vi "Gas_Release_Control.vi"(5 "Extra Commands":string, 6 "Density Ratio":string="Carrier 1 only", 7 "Strength (% by volume)":dbl format="%.3f", 8 "Stack flowrate (l/min)":dbl format="%.2f", 9 "Source Status":T2) -> (0 "error out":errorcluster, 1 "Flowrates (kg/min)":dbl[](array[numeric]) format="%.2f", 2 "Source Est Time (s)":dbl, 3 "Flowrates Achieved?":bool)   [LabVIEW 2012]
uses:
  ADAM Controls/Client_Source_Status.ctl
  ADAM Controls/Client_Source.ctl
  ADAM Controls/Channel_names.ctl
  ADAM Controls/Module_type_ADAM.ctl
  ADAM Controls/Calib_type_ADAM.ctl
  ADAM Controls/Channel_State.ctl
  ADAM Controls/Ch_description_ADAM.ctl
  ADAM Controls/Function_ADAM.ctl
  ADAM Controls/Address.ctl
  ADAM Controls/Update_scan_value.ctl
  Anemometry/Anemometry Sub Vis/Controls/In_Range.ctl
  Anemometry/Anemometry Sub Vis/Globals/Preference_global.vi
  Anemometry/Anemometry Sub Vis/Globals/Extra_Commands_Global.vi
panel:
  out "Error String":string
  out "Currently on":T1=enum."Get Source Clients"
  out "Status of other Clients":string[](array[string])
  out "Source already correct?":bool
  out "No Other Clients are Using Source?":bool
  out "Source Clients":string[](array[string])
  # "-Carrier 1 only\n-Carrier 2 only\n-Enter Ratio"
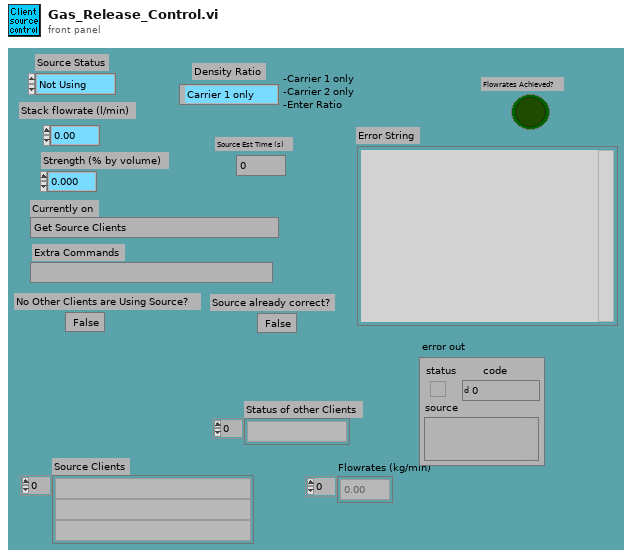
[diagram p1: front panel]
types:
  T1 = typedef "Client_Source.ctl" = enum16{"Start", "Get Source Clients", "Has this client liberty to control the source?", "Declare not using, other client already waiting", "Is the Source already correct?", "Declare waiting, other client is still using", "Control Hi-Tec", "Were the Hi-tecs able to achieve the flowrates?", "Declare source status", "Wait for source to Establish"}
  T2 = typedef "Client_Source_Status.ctl" = enum16{"Not Using", "Using", "Must Have"}
  T3 = typedef "Channel_names.ctl" = enum16{"Active Only", "Active + Off", "All Channels"}
  T4 = typedef "Ch_description_ADAM.ctl" = cluster{"Ch Name":string, "Type":T5, "Function":T6, "Ch State":T7, "Calibration type":T8, "A":dbl, "B":dbl, "C":dbl, "D":dbl, "Comments":string, "Address":T9, "String":string, "Duty":u16}
  T5 = typedef "Module_type_ADAM.ctl" = string
  T6 = typedef "Function_ADAM.ctl" = enum16{"Analogue Input", "Digital Input", "Event counter", "Event rate", "Analogue Output", "Digital Output", "Relay Output"}
  T7 = typedef "Channel_State.ctl" = enum16{"On", "Off", "Always On", "Always Off"}
  T8 = typedef "Calib_type_ADAM.ctl" = enum16{"Raw", "Bx + A", "Cx^2 + Bx + A", "Dx^3 + Cx^2 + Bx + A", "In Band", "Hi-Tec Q", "Hi-Tec M_dot", "Text"}
  T9 = typedef "Address.ctl" = cluster{"Main":i32, "Ch.":i32, "Sub":i32, "Port Name":string}
  T10 = typedef "Update_scan_value.ctl" = cluster{"Channel Name":string, "New Value":dbl}
  T11 = typedef "In_Range.ctl" = enum16{"%", "±", "% & ±"}
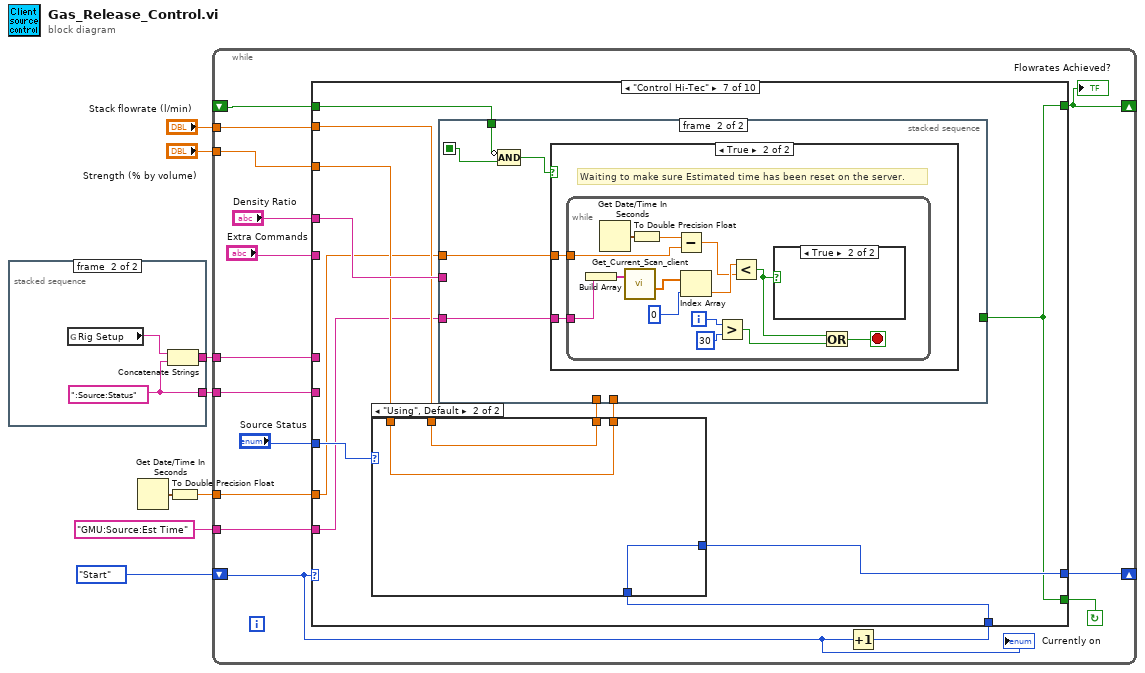
[diagram p0: block diagram]
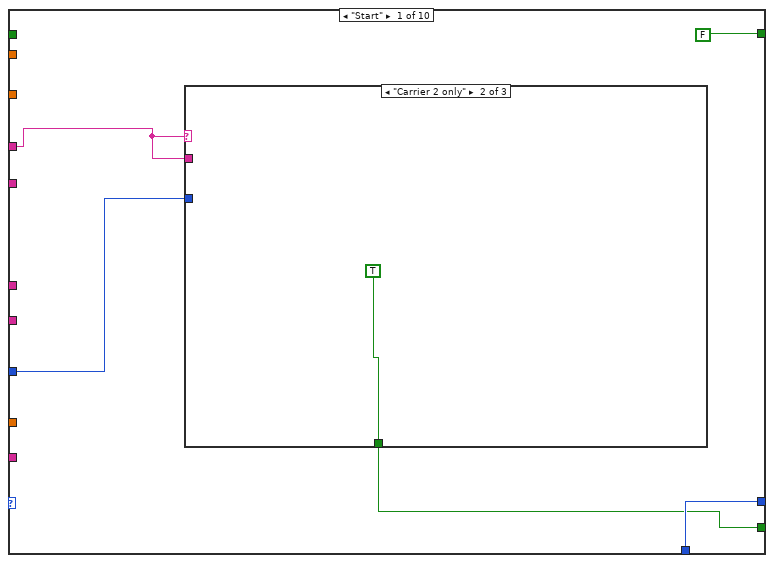
[diagram p2: hidden frame]
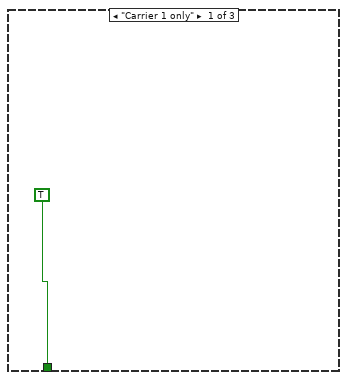
[diagram p3: hidden frame]
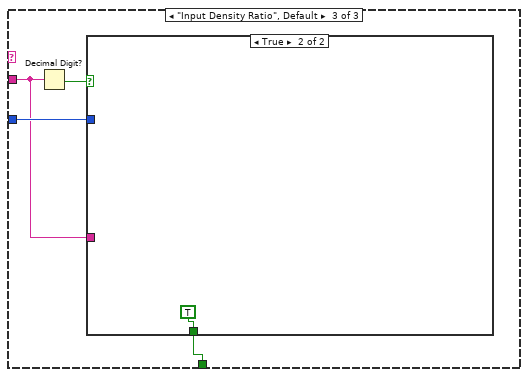
[diagram p4: hidden frame]
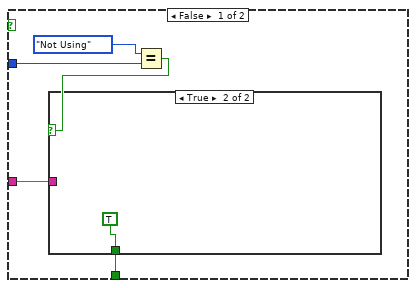
[diagram p5: hidden frame]
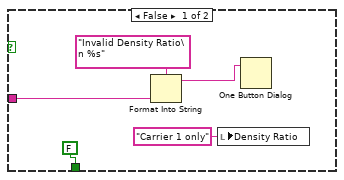
[diagram p6: hidden frame]
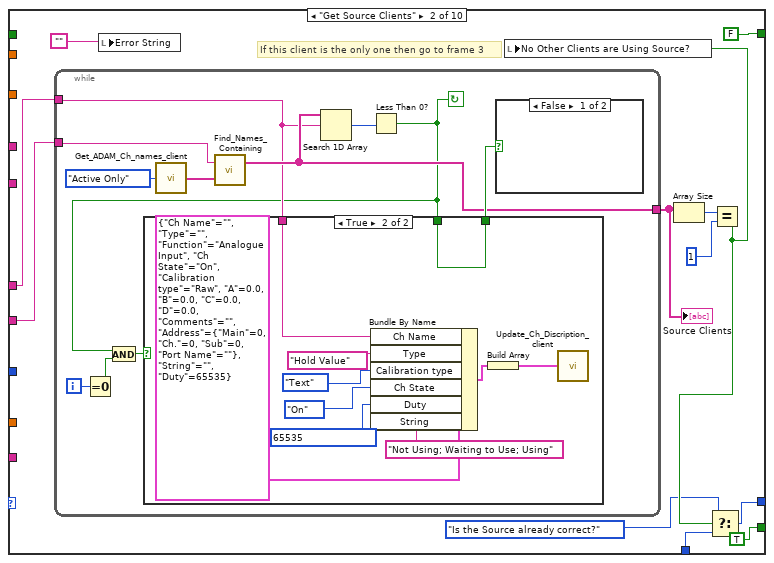
[diagram p7: hidden frame]
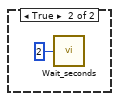
[diagram p8: hidden frame]
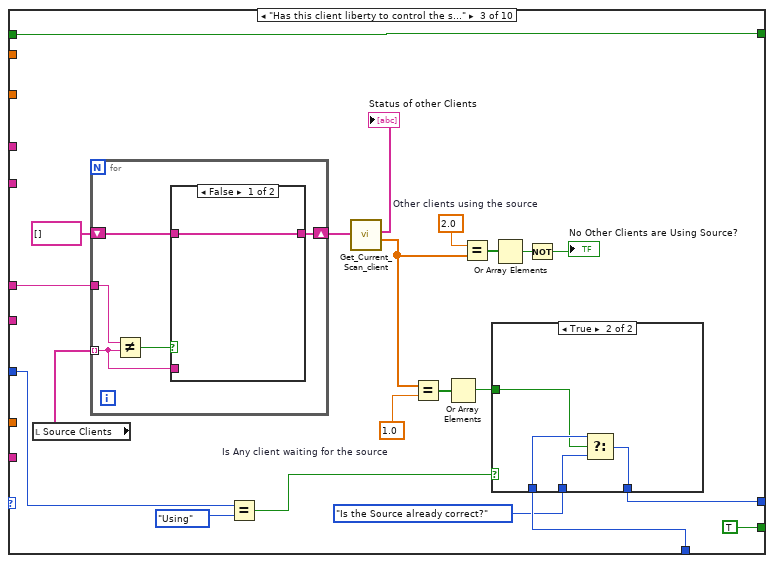
[diagram p10: hidden frame]
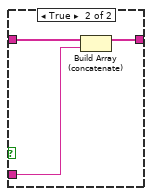
[diagram p12: hidden frame]
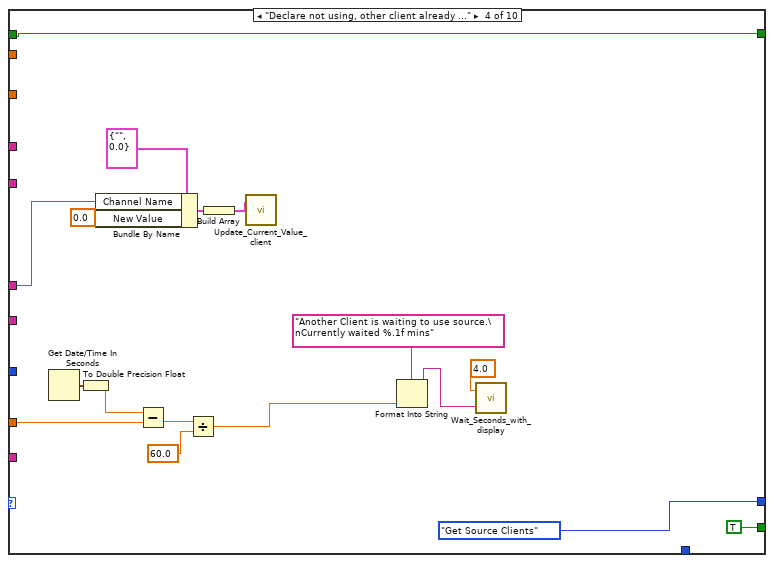
[diagram p13: hidden frame]
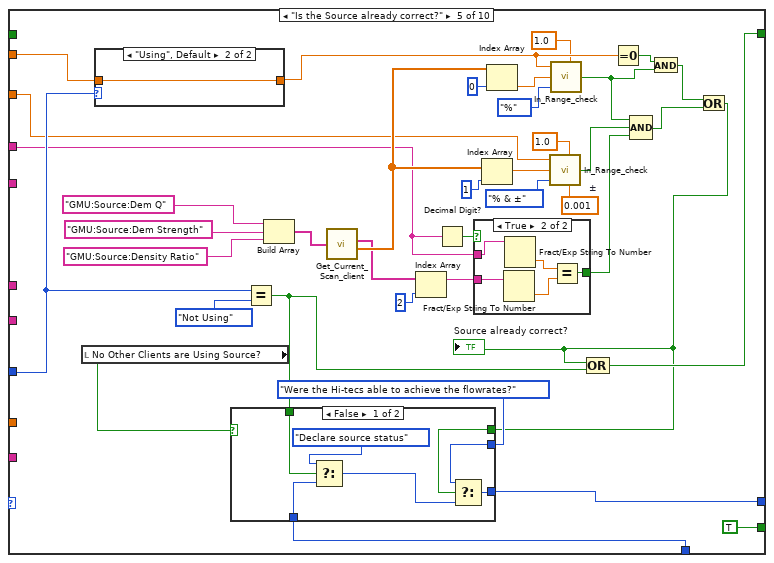
[diagram p14: hidden frame]
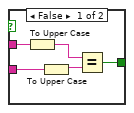
[diagram p15: hidden frame]
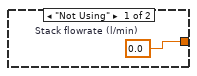
[diagram p16: hidden frame]
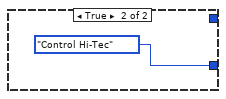
[diagram p17: hidden frame]
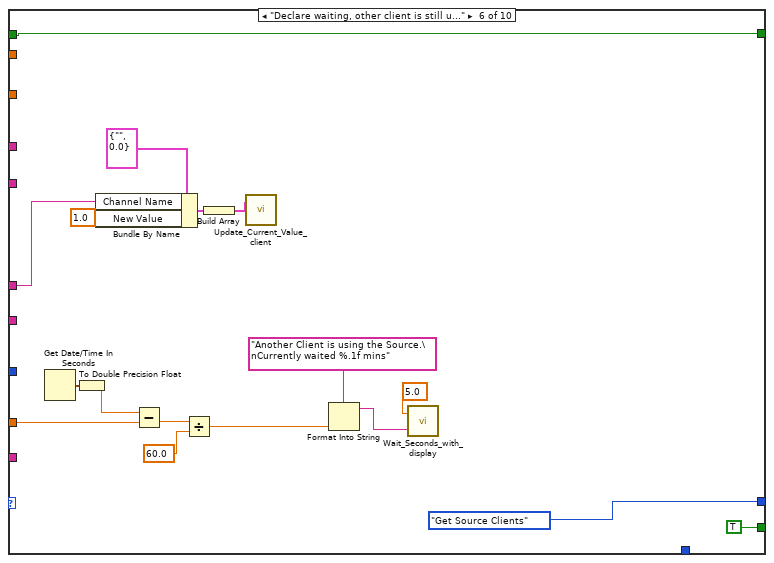
[diagram p18: hidden frame]
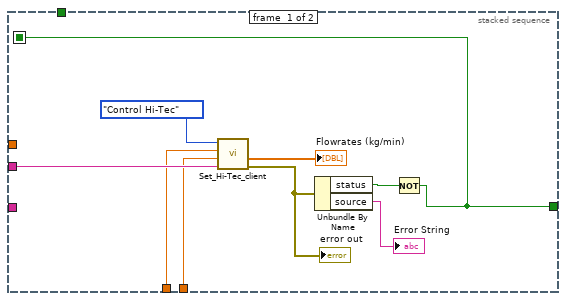
[diagram p19: hidden frame]
diagram:
  n1 = stacked-sequence {
    tunnel: [_ w11] -> w8
    tunnel: [_ w10] -> w7
    frame #0 {
      n2 = call "Run_EnFlo_Hub.vi"() -> ()  [unwired: 8 out]
    }
    frame #1 {
      w11 = ":Source:Status"
      n3 = global read "Preference_global.vi" "Rig Setup"() -> (w9:string)
      n4 = Concatenate Strings(w9, w11) -> (w10:string)
    }
  }
  n5 = Get Date/Time In Seconds() -> (seconds since 1Jan1904=w2:timestamp)
  n6 = To Double Precision Float(number=w2) -> (double precision float=w6:dbl)
  n7 = while {
    tunnel: w6 -> [w22]
    tunnel: w7 -> [w25]
    shift-left: Client_Source."Start" -> [w20]
    shift-right: [w21] -> _
    tunnel: w8 -> [w26]
    tunnel: "Stack flowrate (l/min)" -> [w16]
    tunnel: "Strength (% by volume)" -> [w15]
    shift-right: [w13] -> _
    shift-left: _ -> [w14]
    tunnel: "GMU:Source:Est Time" -> [w12]
    stop <- w24 continue-if-true
    n8 = Increment(x=w20) -> (x+1=w23:T1)
    n9 = case shown="\"Control Hi-Tec\"" w20 {
      tunnel: w16 -> [_ _ _ _ w167 _ w220 w265 _ w313]
      tunnel: w15 -> [_ _ _ _ w150 _ w218 _ _ _]
      tunnel: "Density Ratio" -> [w30 _ _ _ w142 _ w223 _ _ _]
      tunnel: w26 -> [_ w61 _ _ _ _ _ _ _ _]
      tunnel: [w31 w57 w98 Client_Source."Get Source Clients" w138 Client_Source."Get Source Clients" w217 w267 w303 w319] -> w21
      tunnel: w25 -> [_ w60 w105 w131 _ w206 _ _ w309 _]
      tunnel: [w29 TRUE TRUE TRUE TRUE TRUE w213 TRUE TRUE FALSE] -> w24
      tunnel: w23 -> [w31 w56 w100 _ w168 _ w216 w266 w303 w319]
      tunnel: w22 -> [_ _ _ w129 _ w201 w214 _ _ _]
      tunnel: "Source Status" -> [w28 _ w89 _ w159 _ w222 w264 w307 w318]
      tunnel: "Extra Commands" -> [_ _ _ _ _ _ _ _ _ w316]
      tunnel: [FALSE FALSE w85 w121 w140 w196 w213 w263 w301 w314] -> w13
      tunnel: w14 -> [_ _ w85 w121 _ w196 w212 _ w301 w314]
      tunnel: w12 -> [_ _ _ _ _ _ w215 w261 _ _]
      frame "Start" {
        n10 = case shown="\"Carrier 2 only\"" w30 {
          tunnel: w30 -> [_ _ w34]
          tunnel: [TRUE TRUE w35] -> w29
          tunnel: w28 -> [_ _ w36]
          frame "Carrier 1 only" {
            (unwired) TRUE
            (unwired) 0.0 ("Qc2")
          }
          frame "Carrier 2 only" {
            (unwired) TRUE
            (unwired) 0.0 ("Qc1")
          }
          frame "Input Density Ratio", Default {
            n11 = Decimal Digit?(1:w34) -> (0:w37:bool)
            n12 = case shown="True" w37 {
              tunnel: w36 -> [w41 _]
              tunnel: [w39 TRUE] -> w35
              tunnel: w34 -> [w38 _]
              frame False {
                n13 = Equal?(x=Client_Source_Status."Not Using" ("Source Status"), y=w41) -> (x = y?=w40:bool)
                n14 = case shown="True" w40 {
                  tunnel: [FALSE TRUE] -> w39
                  tunnel: w38 -> [w46 _]
                  frame False {
                    n15 = Format Into String(format string="Invalid Density Ratio\n %s", w46) -> (resulting string=w44:string)  [unwired: 2 in, 1 out]
                    n16 = local write "Density Ratio"("Carrier 1 only" ("Density Ratio")) -> ()
                    n17 = One Button Dialog(message=w44) -> ()  [unwired: 2 out]
                  }
                  frame True {
                  }
                }
              }
              frame True {
              }
            }
          }
        }
      }
      frame "Get Source Clients" {
        # "If this client is the only one then go to frame 3"
        n18 = while {
          tunnel: [w65] -> w54
          tunnel: w60 -> [w64]
          tunnel: w61 -> [w72]
          i -> [w69]
          stop <- w62 continue-if-true
          n19 = Equal To 0?(x=w69) -> (x = 0?=w68:bool)
          n20 = call "Get_ADAM_Ch_names_client.vi"("Channel names set"=Channel_names."Active Only") -> ("Ch names"=w70:string[])
          n21 = call "Find_Names_Containing.vi"("Ch names"=w70, "String to match"=w72) -> ("Matched Names"=w65:string[])  [unwired: 1 out]
          n22 = Search 1D Array(1D array=w65, element=w64) -> (index of element=w63:i32)  [unwired: 1 out]
          n23 = Less Than 0?(x=w63) -> (x < 0?=w62:bool)
          n24 = And(x=w62, y=w68) -> (x .and. y?=w67:bool)
          n25 = case shown="True" w67 {
            tunnel: w64 -> [_ w81]
            tunnel: [w74 w77] -> w66
            tunnel: w62 -> [w74 w77]
            frame False {
            }
            frame True {
              n26 = Bundle By Name(cluster=T4 {"Ch Name"="", "Type"="", "Function"=enum."Analogue Input", "Ch State"=enum."On", "Calibration type"=enum."Raw", "A"=0.0, "B"=0.0, "C"=0.0, "D"=0.0, "Comments"="", "Address"={"Main"=0, "Ch."=0, "Sub"=0, "Port Name"=""}, "String"="", "Duty"=65535} ("Ch Discription"), "Ch Name"=w81, "Type"=T5 "Hold Value", "Calibration type"=Calib_type_ADAM."Text", "Ch State"=Channel_State."On", "Duty"=u16 65535 ("Bundle Element"), "String"="Not Using; Waiting to Use; Using") -> (w79:T4)
              n27 = Build Array(w79) -> (w78:T4[])
              n28 = call "Update_Ch_Discription_client.vi"("Channels to update In"=w78) -> ()  [unwired: 1 out]
            }
          }
          n29 = case shown="False" w66 {
            frame False {
            }
            frame True {
              n30 = call "Wait_seconds.vi"("Seconds to wait"=u32 2) -> ()
            }
          }
        }
        "Source Clients" <- w54
        n31 = local write "Error String"("") -> ()
        n32 = Array Size(array=w54) -> (size(s)=w59:i32)
        n33 = Equal?(x=w59, y=1) -> (x = y?=w53:bool)
        n34 = local write "No Other Clients are Using Source?"(w53) -> ()
        n35 = Select(t=Client_Source."Is the Source already correct?", s=w53, f=w56) -> (s? t:f=w57:T1)
      }
      frame "Has this client liberty to control the source?" {
        w97 = 2.0  # Other clients using the source
        w103 = 1.0  # Is Any client waiting for the source
        n36 = local read "Source Clients"() -> (w99:string[])
        n37 = for {
          tunnel: w99 -> [w111] mode=indexing
          tunnel: w105 -> [w115]
          shift-right: [w112] -> w95
          shift-left: string[] [] -> [w113]
          n38 = Not Equal?(x=w115, y=w111) -> (x != y?=w114:bool)
          n39 = case shown="False" w114 {
            tunnel: w113 -> [w116 w119]
            tunnel: [w116 w118] -> w112
            tunnel: w111 -> [_ w117]
            frame False {
            }
            frame True {
              n40 = Build Array (concatenate)(w119, w117) -> (w118:string[])
            }
          }
        }
        n41 = Equal?(x=w89, y=Client_Source_Status."Using" ("Source Status")) -> (x = y?=w88:bool)
        n42 = call "Get_Current_Scan_client.vi"("ADAM Ch Names"=w95) -> ("String values"=→"Status of other Clients":string[], "Numerical Values"=w92:dbl[])  [unwired: 2 out]
        n43 = Equal?(x=w92, y=w103) -> (x = y?=w102:bool[])
        n44 = Or Array Elements(Boolean array=w102) -> (logical OR=w93:bool)
        n45 = Equal?(x=w97, y=w92) -> (x = y?=w96:bool[])
        n46 = case shown="True" w88 {
          tunnel: w100 -> [_ w110]
          tunnel: [w106 w109] -> w98
          tunnel: w93 -> [_ w108]
          tunnel: Client_Source."Is the Source already correct?" -> [w106 w107]
          frame False {
          }
          frame True {
            n47 = Select(t=w110, s=w108, f=w107) -> (s? t:f=w109:T1)
          }
        }
        n48 = Or Array Elements(Boolean array=w96) -> (logical OR=w91:bool)
        n49 = Not(x=w91) -> (.not. x?=→"No Other Clients are Using Source?":bool)
      }
      frame "Declare not using, other client already waiting" {
        n50 = Get Date/Time In Seconds() -> (seconds since 1Jan1904=w120:timestamp)
        n51 = To Double Precision Float(number=w120) -> (double precision float=w130:dbl)
        n52 = Bundle By Name(cluster=T10 {"Channel Name"="", "New Value"=0.0} ("Update Scan Value Cluster"), "Channel Name"=w131, "New Value"=0.0 ("Bundle Element")) -> (w134:T10)
        n53 = Subtract(x=w130, y=w129) -> (x-y=w128:dbl)
        n54 = Divide(x=w128, y=60.0) -> (x/y=w122:dbl)
        n55 = Build Array(w134) -> (w133:T10[])
        n56 = call "Update_Current_Value_client.vi"("Update array in"=w133) -> ()  [unwired: 1 in]
        n57 = Format Into String(format string="Another Client is waiting to use source.\nCurrently waited %.1f mins" ("Format String"), w122) -> (resulting string=w125:string)  [unwired: 2 in, 1 out]
        n58 = call "Wait_Seconds_with_display.vi"("Message"=w125, "Seconds to wait"=4.0) -> ()  [unwired: 2 out]
      }
      frame "Is the Source already correct?" {
        w147 = 0.001  # ±
        n59 = local read "No Other Clients are Using Source?"() -> (w169:bool)
        n60 = case shown="\"Using\", Default" w159 {
          tunnel: [w185 w186] -> w157
          tunnel: w167 -> [_ w186]
          frame "Not Using" {
            w185 = 0.0  # Stack flowrate (l/min)
          }
          frame "Using", Default {
          }
        }
        n61 = Equal?(x=w159, y=Client_Source_Status."Not Using" ("Source Status")) -> (x = y?=w158:bool)
        n62 = Build Array("GMU:Source:Dem Q", "GMU:Source:Dem Strength", "GMU:Source:Density Ratio") -> (w171:string[])
        n63 = call "Get_Current_Scan_client.vi"("ADAM Ch Names"=w171) -> ("String values"=w144:string[], "Numerical Values"=w164:dbl[])  [unwired: 2 out]
        n64 = Index Array(array=w144, index=2 ("Index")) -> (element=w143:string)
        n65 = Decimal Digit?(1:w142) -> (0:w146:bool)
        n66 = case shown="True" w146 {
          tunnel: [w178 w181] -> w141
          tunnel: w142 -> [w177 w183]
          tunnel: w143 -> [w176 w184]
          frame False {
            n67 = To Upper Case(1:w177) -> (0:w179:string)
            n68 = To Upper Case(1:w176) -> (0:w175:string)
            n69 = Equal?(x=w179, y=w175) -> (x = y?=w178:bool)
          }
          frame True {
            n70 = Fract/Exp String To Number(string=w184) -> (number=w180:dbl)  [unwired: 4 out]
            n71 = Fract/Exp String To Number(string=w183) -> (number=w182:dbl)  [unwired: 4 out]
            n72 = Equal?(x=w182, y=w180) -> (x = y?=w181:bool)
          }
        }
        n73 = Index Array(array=w164, index=1 ("Index")) -> (element=w149:dbl)
        n74 = Index Array(array=w164, index=0 ("Index")) -> (element=w156:dbl)
        n75 = call "In_Range_check.vi"("±"=w147, "%"=1.0, "Mode"=In_Range."% & ±", "Value"=w149, "Setpoint"=w150) -> ("In Range"=w148:bool)  [unwired: 2 out]
        n76 = call "In_Range_check.vi"("%"=1.0, "Mode"=In_Range."%", "Value"=w156, "Setpoint"=w157) -> ("In Range"=w155:bool)  [unwired: 1 in, 2 out]
        n77 = Equal To 0?(x=w157) -> (x = 0?=w163:bool)
        n78 = Compound Arithmetic op=AND(w155, w148, w141) -> (w161:bool)
        n79 = And(x=w163, y=w155) -> (x .and. y?=w162:bool)
        n80 = Or(x=w162, y=w161) -> (x .or. y?=w137:bool)
        "Source already correct?" <- w137
        n81 = case shown="False" w169 {
          tunnel: w168 -> [w193 _]
          tunnel: w158 -> [w192 _]
          tunnel: w137 -> [w190 _]
          tunnel: Client_Source."Were the Hi-tecs able to achieve the flowrates?" -> [w188 _]
          tunnel: [w187 Client_Source."Control Hi-Tec"] -> w138
          frame False {
            n82 = Select(t=Client_Source."Declare source status", s=w192, f=w193) -> (s? t:f=w189:T1)
            n83 = Select(t=w188, s=w190, f=w189) -> (s? t:f=w187:T1)
          }
          frame True {
          }
        }
        n84 = Compound Arithmetic op=OR(w137, w158) -> (w140:bool)
      }
      frame "Declare waiting, other client is still using" {
        n85 = Get Date/Time In Seconds() -> (seconds since 1Jan1904=w195:timestamp)
        n86 = To Double Precision Float(number=w195) -> (double precision float=w204:dbl)
        n87 = Bundle By Name(cluster=T10 {"Channel Name"="", "New Value"=0.0} ("Update Scan Value Cluster"), "Channel Name"=w206, "New Value"=1.0 ("Bundle Element")) -> (w209:T10)
        n88 = Subtract(x=w204, y=w201) -> (x-y=w203:dbl)
        n89 = Divide(x=w203, y=60.0) -> (x/y=w197:dbl)
        n90 = Build Array(w209) -> (w208:T10[])
        n91 = call "Update_Current_Value_client.vi"("Update array in"=w208) -> ()  [unwired: 1 in]
        n92 = Format Into String(format string="Another Client is using the Source.\nCurrently waited %.1f mins" ("Format String"), w197) -> (resulting string=w200:string)  [unwired: 2 in, 1 out]
        n93 = call "Wait_Seconds_with_display.vi"("Message"=w200, "Seconds to wait"=5.0) -> ()  [unwired: 2 out]
      }
      frame "Control Hi-Tec" {
        n94 = case shown="\"Using\", Default" w222 {
          tunnel: [w257 w260] -> w221
          tunnel: w220 -> [_ w260]
          tunnel: [w256 w259] -> w219
          tunnel: w218 -> [_ w259]
          tunnel: [Client_Source."Declare source status" w258] -> w217
          tunnel: w216 -> [_ w258]
          frame "Not Using" {
            w256 = 0.0  # Strength (% by volume)
            w257 = 0.0  # Stack flowrate (l/min)
          }
          frame "Using", Default {
          }
        }
        n95 = stacked-sequence {
          seq-local: [w224 _] -> [_ w235]
          tunnel: w223 -> [w231 _]
          tunnel: w221 -> [w229 _]
          tunnel: w219 -> [w228 _]
          tunnel: w215 -> [_ w237]
          tunnel: w214 -> [_ w236]
          tunnel: [w224 _] -> w213
          tunnel: w212 -> [_ w234]
          frame #0 {
            n96 = call "Set_Hi-Tec_client.vi"("Density Ratio"=w231, "Strength (% by volume)"=w228, "Stack flowrate (l/min)"=w229, "Mode"=enum16{"Control Hi-Tec", "Check Hi-Tec Demands"}."Control Hi-Tec") -> ("error out"=w227:errorcluster, "Flowrates (kg/min)"=→"Flowrates (kg/min)":dbl[])  [unwired: 1 in, 3 out]
            "error out" <- w227
            n97 = Unbundle By Name(w227) -> ("status"=w225:bool, "source"=→"Error String":string)
            n98 = Not(x=w225) -> (.not. x?=w224:bool)
          }
          frame #1 {
            n99 = Compound Arithmetic op=AND(invert w234, w235) -> (w233:bool)
            n100 = case shown="True" w233 {
              tunnel: w237 -> [_ w239]
              tunnel: w236 -> [_ w238]
              frame False {
              }
              frame True {
                # "Waiting to make sure Estimated time has been reset on the server."
                n101 = while {
                  tunnel: w239 -> [w252]
                  tunnel: w238 -> [w247]
                  i -> [w244]
                  stop <- w240 stop-if-true
                  n102 = Build Array(w252) -> (w253:string[])
                  n103 = Get Date/Time In Seconds() -> (seconds since 1Jan1904=w249:timestamp)
                  n104 = call "Get_Current_Scan_client.vi"("ADAM Ch Names"=w253) -> ("Numerical Values"=w251:dbl[])  [unwired: 3 out]
                  n105 = To Double Precision Float(number=w249) -> (double precision float=w248:dbl)
                  n106 = Subtract(x=w248, y=w247) -> (x-y=w245:dbl)
                  n107 = Index Array(array=w251, index=0) -> (element=w246:dbl)
                  n108 = Greater?(x=w244, y=30) -> (0:w241:bool)
                  n109 = Less?(x=w246, y=w245) -> (x < y?=w242:bool)
                  n110 = case shown="True" w242 {
                    frame False {
                      n111 = Wait (ms)(milliseconds to wait=u32 1000) -> ()  [unwired: 1 out]
                    }
                    frame True {
                    }
                  }
                  n112 = Or(x=w242, y=w241) -> (x .or. y?=w240:bool)
                }
              }
            }
          }
        }
      }
      frame "Were the Hi-tecs able to achieve the flowrates?" {
        n113 = Get Date/Time In Seconds() -> (seconds since 1Jan1904=w262:timestamp)
        n114 = To Double Precision Float(number=w262) -> (double precision float=w269:dbl)
        n115 = while {
          tunnel: w264 -> [w277]
          tunnel: w265 -> [w275]
          tunnel: [w273] -> w268
          tunnel: w269 -> [w290]
          tunnel: [w273] -> w263
          tunnel: w261 -> [w271]
          stop <- w286 continue-if-true
          w274 = 0.1  # ±
          w282 = 1.0  # %
          n116 = case shown="\"Using\", Default" w277 {
            tunnel: [w295 w296] -> w276
            tunnel: w275 -> [_ w296]
            frame "Not Using" {
              w295 = 0.0  # Stack flowrate (l/min)
            }
            frame "Using", Default {
            }
          }
          n117 = Get Date/Time In Seconds() -> (seconds since 1Jan1904=w272:timestamp)
          n118 = To Double Precision Float(number=w272) -> (double precision float=w291:dbl)
          n119 = Subtract(x=w291, y=w290) -> (x-y=w289:dbl)
          n120 = Build Array("GMU:Source:Dem Q", w271) -> (w294:string[])
          n121 = Less?(x=w289, y=120.0) -> (x < y?=w287:bool)
          n122 = call "Get_Current_Scan_client.vi"("ADAM Ch Names"=w294) -> ("Numerical Values"=w280:dbl[])  [unwired: 3 out]
          n123 = Index Array(array=w280, index=1 ("Index")) -> (element=w292:dbl)
          "Source Est Time (s)" <- w292
          n124 = Index Array(array=w280, index=0 ("Index")) -> (element=w284:dbl)
          n125 = Greater Than 0?(x=w292) -> (x > 0?=w278:bool)
          n126 = call "In_Range_check.vi"("±"=w274, "%"=w282, "Mode"=In_Range."% & ±", "Value"=w284, "Setpoint"=w276) -> ("In Range"=w279:bool)  [unwired: 2 out]
          n127 = And(x=w279, y=w278) -> (x .and. y?=w273:bool)
          n128 = Compound Arithmetic op=AND(invert w273, w287) -> (w286:bool)
          n129 = case shown="True" w286 {
            frame False {
            }
            frame True {
              n130 = Wait (ms)(milliseconds to wait=u32 1000) -> ()  [unwired: 1 out]
            }
          }
        }
        n131 = case shown="True" w268 {
          tunnel: [Client_Source."Control Hi-Tec" w300] -> w267
          tunnel: w266 -> [_ w300]
          frame False {
            n132 = local write "Source Status"(Client_Source_Status."Not Using" ("Source Status")) -> ()
          }
          frame True {
          }
        }
      }
      frame "Declare source status" {
        n133 = case shown="\"Using\"" w307 {
          tunnel: [0.0 2.0 2.0] -> w302
          frame "Not Using" {
          }
          frame "Using" {
          }
          frame "Must Have" {
          }
        }
        n134 = Bundle By Name(cluster=T10 {"Channel Name"="", "New Value"=0.0} ("Update Scan Value Cluster"), "Channel Name"=w309, "New Value"=w302) -> (w305:T10)
        n135 = Build Array(w305) -> (w304:T10[])
        n136 = call "Update_Current_Value_client.vi"("Update array in"=w304) -> ()  [unwired: 1 in]
      }
      frame "Wait for source to Establish" {
        n137 = Not Equal?(x=Client_Source_Status."Not Using" ("Source Status"), y=w318) -> (x != y?=w315:bool)
        n138 = case shown="True" w315 {
          tunnel: w316 -> [_ w337]
          tunnel: w313 -> [_ w326]
          frame False {
          }
          frame True {
            n139 = global read "Extra_Commands_Global.vi" "Establish Exp Conditions (s)"() -> (w338:string)
            n140 = global read "Preference_global.vi" "Default Source Establishment Time (s)"() -> (w329:dbl)
            n141 = Equal To 0?(x=w326) -> (x = 0?=w324:bool)
            n142 = Divide(x=100.0, y=w326) -> (x/y=w323:dbl)
            n143 = local read "Source Est Time (s)"() -> (w330:dbl)
            n144 = Not A Number/Path/Refnum?(number/path/refnum=w330) -> (NaN/Path/Refnum?=w334:bool)
            n145 = call "Extra_Commands.vi"("String to Search"=w337, "Command"=w338) -> ("Numeric Value"=w331:dbl, "Command Found"=w332:bool)  [unwired: 1 in, 3 out]
            n146 = Select(t=w331, s=w332, f=w329) -> (s? t:f=w328:dbl)
            n147 = Select(t=0.0, s=w324, f=w323) -> (s? t:f=w321:dbl)
            n148 = Add(x=w321, y=w328) -> (x+y=w327:dbl)
            n149 = Subtract(x=w327, y=w330) -> (x-y=w333:dbl)
            n150 = Greater Than 0?(x=w333) -> (x > 0?=w336:bool)
            n151 = Or(x=w336, y=w334) -> (x .or. y?=w335:bool)
            n152 = case shown="True" w335 {
              tunnel: w334 -> [_ w342]
              tunnel: w327 -> [_ w341]
              tunnel: w333 -> [_ w340]
              frame False {
              }
              frame True {
                n153 = Select(t=w341, s=w342, f=w340) -> (s? t:f=w339:dbl)
                n154 = call "Wait_Seconds_with_display.vi"("Message"="Establishing Source", "Seconds to wait"=w339) -> ()  [unwired: 2 out]
              }
            }
          }
        }
      }
    }
    "Flowrates Achieved?" <- w13
    "Currently on" <- w20
  }
